vi "Do.vi"(8 "error in (no error)":errorcluster, 10 "Actor in":refnum<class "Actor.lvclass">, 11 "Display Results":refnum<class "Display Results.lvclass">) -> (0 "error out":errorcluster, 2 "Actor out":refnum<class "Actor.lvclass">)   [LabVIEW 2017, in "Measurement UI.lvlib" / "Display Results.lvclass"]
uses:
  Display Results.lvclass
  <vilib>/ActorFramework/Actor/Actor.lvclass
  Msmt UI/Measurement UI.lvclass
  C:/Program Files (x86)/National Instruments/LabVIEW 2017/vi.lib/ActorFramework/Actor/Actor.lvclass
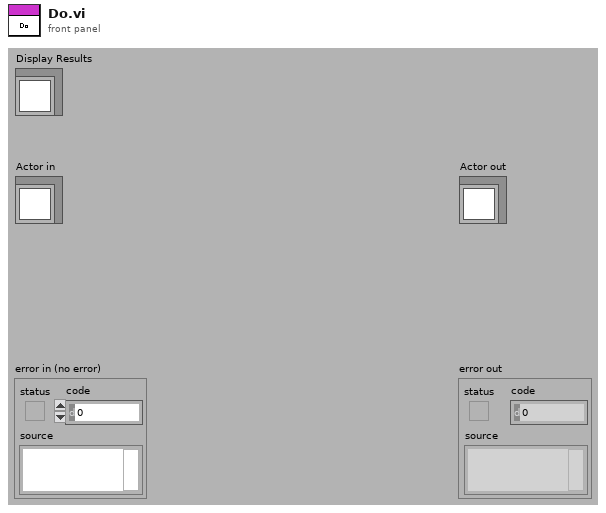
[diagram p1: front panel]
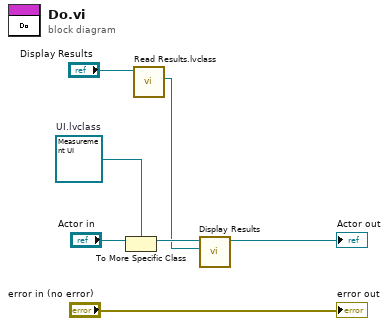
[diagram p0: block diagram]
diagram:
  w6 = refnum<class "Measurement UI.lvclass"> refnum  # UI.lvclass
  n1 = To More Specific Class(target class=w6, reference="Actor in") -> (specific class reference=w4:refnum<class "Measurement UI.lvclass">)  [unwired: 1 in, 1 out]
  n2 = call "Read Results.lvclass.vi"("Display Results in"="Display Results") -> ("Results.lvclass"=w1:refnum<class "Results.lvclass">)  [unwired: 8 in, 2 out]
  n3 = call-dynamic "Display Results.vi"("Results.lvclass"=w1, "Operator UI in"=w4) -> ("Operator UI out"=→"Actor out":refnum<class "Measurement UI.lvclass">)  [unwired: 8 in, 1 out]
  "error out" <- "error in (no error)"
